vi "Get Probe Angle-Offset-Range.vi"(11 "Probe Select":i32) -> (0 "Probe Offset":sgl, 1 "Angle":sgl, 2 "Meas. Range":sgl, 3 "Name":string)   [LabVIEW 2015, in "Tool Cfg.lvlib"]
uses:
  Tool Cfg.lvlib
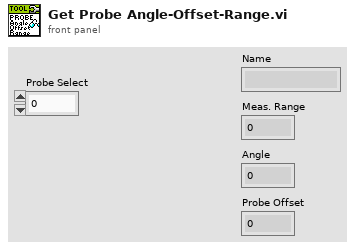
[diagram p1: front panel]
types:
  T1 = typedef "Tool Cfg.lvlib/_ProbeConfigParams Cluster--typedef.ctl" = cluster{"Name":string, "Laser Init Pwr":u16, "Laser Gain":u8, "Integ Count":u16, "Meas. Range":sgl, "Angle":sgl, "Probe Offset":sgl, "Sensor Block":T2}
  T2 = typedef "Tool Cfg.lvlib/_Sensor Block Cluster--typedef.ctl" = cluster{"nSensors":u16, "SensorCfgParams Array":T3[]}
  T3 = typedef "Tool Cfg.lvlib/_SensorConfigParams Cluster--typedef.ctl" = cluster{"Total Pixels":u16, "Positive  Peaks":bool, "CalibrCoefArray":dbl[], "Start Idx":u16, "End Idx":u16}
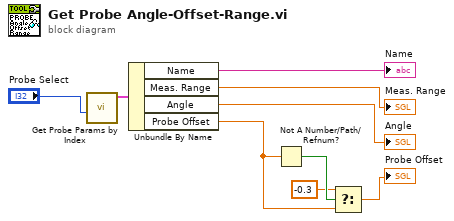
[diagram p0: block diagram]
diagram:
  n1 = call "Get Probe Params by Index.vi"("Probe Select"="Probe Select") -> ("Probe Cfg Params"=w9:T1)  [unwired: 10 in]
  n2 = Unbundle By Name(w9) -> ("Name"=→"Name":string, "Meas. Range"=→"Meas. Range":sgl, "Angle"=→"Angle":sgl, "Probe Offset"=w2:sgl)
  n3 = Not A Number/Path/Refnum?(number/path/refnum=w2) -> (NaN/Path/Refnum?=w4:bool)
  n4 = Select(t=-0.3, s=w4, f=w2) -> (s? t:f=→"Probe Offset":dbl)
